vi "get_test_output.vi"(7 "DAQmx Device Name":tag="Dev1", 8 "error in":errorcluster, 10 "Meas environment":T3) -> (0 "error out":errorcluster, 2 "Outputs":T2)   [LabVIEW 2023]
doc: "This VI performs a set of voltage measurements defined in the state machine as follows:\n- get Input V: performs a Measure Vin type measurement and saves the DC/RMS result as Input V avg\n- get Output V: performs a Measure Vout type measurement and saves the DC/RMS result as Output V avg, the Amplitude result as Output V ampl and based on the Rload_value Ohm environmental value calculates the Output Current\n- get Input Current: performs a Measure VRsense type measurement, and based on the ratio of DC/RMS result and the Rsense_value_Ohm environmental value saves the Input current\n- calc Efficency: calculates the input and output powers based on the output and input voltage and current values. As a ratio of output and input power the efficiency value is calculated and saved.\n- disable loads: deactivates the loads (all loads set to FALSE)\n-end"
uses:
  ctl_get_test_output_states_enum.ctl
  ctl_test_outputs_cluster.ctl
  ctl_load_set_cluster.ctl
  ctl_meas_env_cluster.ctl
panel:
  out "Current state":T1
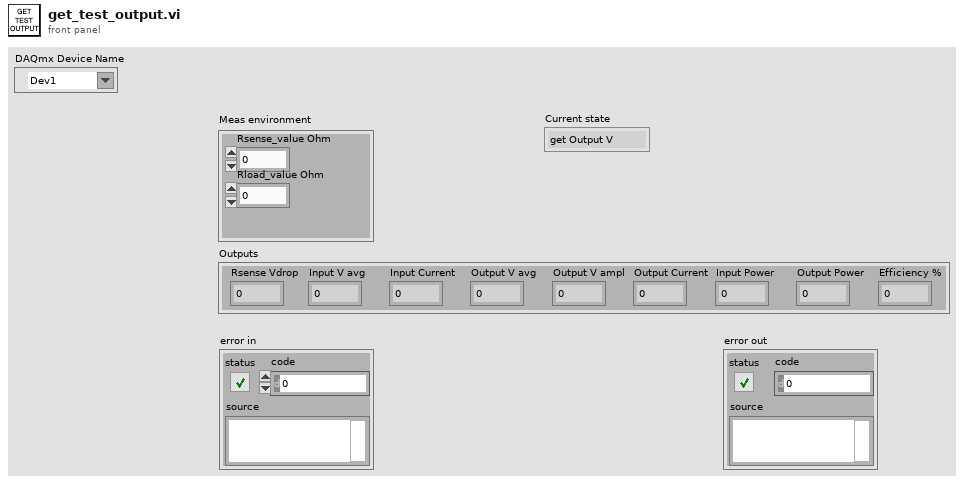
[diagram p1: front panel]
types:
  T1 = typedef "ctl_get_test_output_states_enum.ctl" = enum16{"get Output V", "get Input V", "get Input Current", "calc Efficiency", "disable loads", "end"}
  T2 = typedef "ctl_test_outputs_cluster.ctl" = cluster{"Output V avg":dbl, "Output V ampl":dbl, "Input Current":dbl, "Output Current":dbl, "Efficiency %":dbl, "Input V avg":dbl, "Input Power":dbl, "Output Power":dbl, "Rsense Vdrop":dbl}
  T3 = typedef "ctl_meas_env_cluster.ctl" = cluster{"Rsense_value Ohm":dbl, "Rload_value Ohm":dbl}
  T4 = typedef "ctl_voltage_meas_settings_cluster.ctl" = cluster{"Physical Channel":tag, "Min Voltage":dbl, "Max Voltage":dbl, "Terminal Configuration":i32, "Sample Rate":dbl, "Number of Samples":i32}
  T5 = typedef "ctl_load_set_cluster.ctl" = cluster{"Resistor 1":bool, "Resistor 2":bool, "Resistor 3":bool, "Resistor 4":bool}
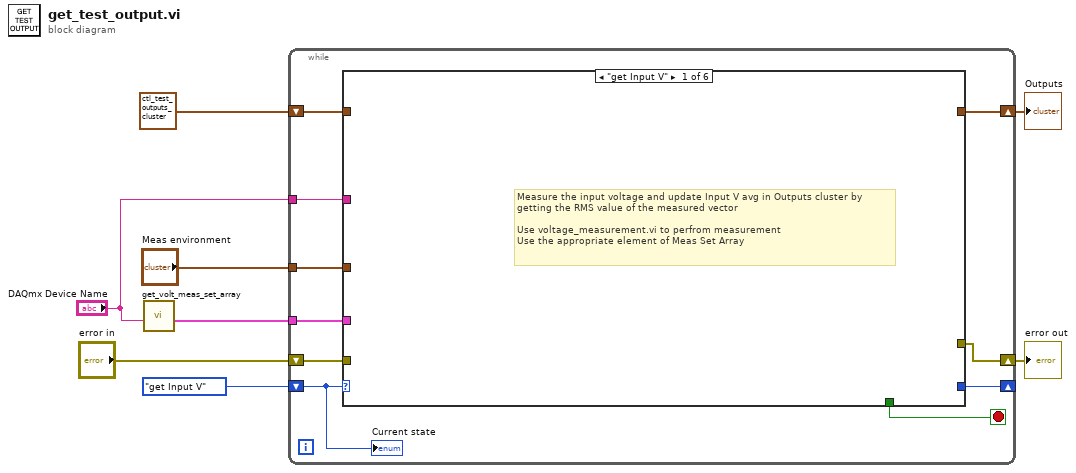
[diagram p0: block diagram]
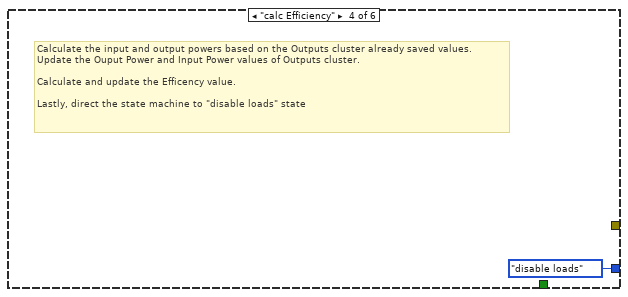
[diagram p4: hidden frame]
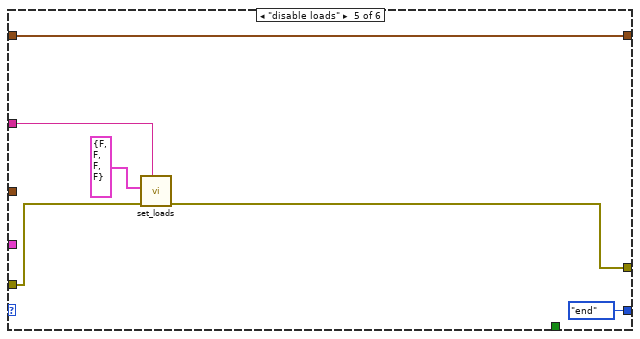
[diagram p5: hidden frame]
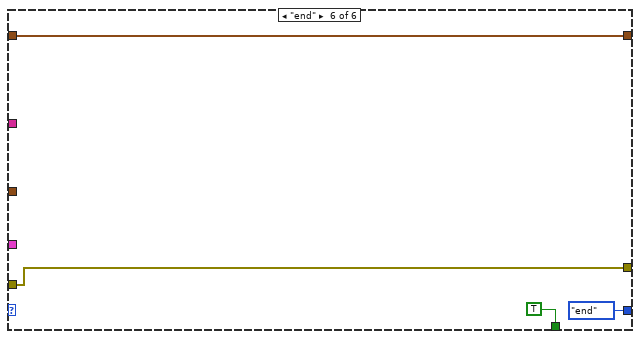
[diagram p6: hidden frame]
diagram:
  n1 = call "get_volt_meas_set_array.vi"("DAQmx Device Name"="DAQmx Device Name") -> ("Voltage meas settings array"=w5:T4[])  [unwired: 10 in]
  n2 = while {
    tunnel: "Meas environment" -> [w17]
    shift-right: [w11] -> _
    shift-left: ctl_get_test_output_states_enum."get Input V" -> [w18]
    shift-right: [w15] -> w3
    shift-left: T2 {"Output V avg"=0.0, "Output V ampl"=0.0, "Input Current"=0.0, "Output Current"=0.0, "Efficiency %"=0.0, "Input V avg"=0.0, "Input Power"=0.0, "Output Power"=0.0, "Rsense Vdrop"=0.0} ("Outputs") -> [w16]
    tunnel: w5 -> [w14]
    shift-right: [w13] -> w2
    shift-left: "error in" -> [w12]
    tunnel: "DAQmx Device Name" -> [w9]
    stop <- w10 stop-if-true
    n3 = case shown="\"get Input V\"" w18 {
      tunnel: w17 -> [_ _ _ _ _ _]
      tunnel: w16 -> [_ _ _ _ w25 w29]
      tunnel: [_ _ _ _ w25 w29] -> w15
      tunnel: w14 -> [_ _ _ _ _ _]
      tunnel: [_ _ _ _ w22 w27] -> w13
      tunnel: w12 -> [_ _ _ _ w23 w27]
      tunnel: [_ _ _ ctl_get_test_output_states_enum."disable loads" ctl_get_test_output_states_enum."end" ctl_get_test_output_states_enum."end"] -> w11
      tunnel: [_ _ _ _ _ TRUE] -> w10
      tunnel: w9 -> [_ _ _ _ w20 _]
      frame "get Input V" {
        # "Measure the input voltage and update Input V avg in Outputs cluster by\ngetting the RMS value of the measured vector\n\nUse voltage_measurement.vi to perfrom measurement\nUse the appropriate element of Meas Set Array"
      }
      frame "get Output V" {
        # "Measure the output voltage and update Output V ampl in Outputs cluster by\ngetting the RMS value of the measured vector.\nUse Ampliutude and Levels waveform fN to get and update Output V ampl in Outputs\nUse Rload_value Ohm from Meas environment cluster to calculate the Output current and\nupdate its value in Outputs cluster\n\nUse voltage_measurement.vi to perfrom measurement\nUse the appropriate element of Meas Set Array"
      }
      frame "get Input Current" {
        # "Measure the differential voltage fall on Rsense resistor and update Input Current in Outputs cluster by\ngetting the RMS value of the measured vector and Rsense_value_Ohm value from the Meas environment cluster.\nUpdate Rsense voltage drop in Output cluster.\n\nUse voltage_measurement.vi to perfrom measurement\nUse the appropriate element of Meas Set Array"
      }
      frame "calc Efficiency" {
        # "Calculate the input and output powers based on the Outputs cluster already saved values.\nUpdate the Ouput Power and Input Power values of Outputs cluster.\n\nCalculate and update the Efficency value.\n\nLastly, direct the state machine to \"disable loads\" state"
      }
      frame "disable loads" {
        n4 = call "set_loads.vi"("DAQmx Device Name"=w20, "error in"=w23, "Load Set"=T5 {"Resistor 1"=FALSE, "Resistor 2"=FALSE, "Resistor 3"=FALSE, "Resistor 4"=FALSE}) -> ("error out"=w22:errorcluster)  [unwired: 8 in]
      }
      frame "end" {
      }
    }
    "Current state" <- w18
  }
  "Outputs" <- w3
  "error out" <- w2
